vi "GetDisplayProperties.vi"(8 "No Error":errorcluster, 11 "Display ID":T2) -> (0 "Error Out":errorcluster, 3 "PropertiesID":T1)   [LabVIEW 2024, in "SDL3.lvlib" / "Video.lvlib"]
doc: "<B>Summary</B>\nGet the properties associated with a display.\n\n<B>Remarks</B>\nThe following read-only properties are provided by SDL:\n\n- <B>SDL_PROP_DISPLAY_HDR_ENABLED_BOOLEAN</B>: true if the display has HDR headroom above the SDR white point. This is for informational and diagnostic purposes only, as not all platforms provide this information at the display level.\n\nOn KMS/DRM:\n- <B>SDL_PROP_DISPLAY_KMSDRM_PANEL_ORIENTATION_NUMBER</B>: the \"panel orientation\" property for the display in degrees of clockwise rotation. Note that this is provided only as a hint, and the application is responsible for any coordinate transformations needed to conform to the requested display orientation."
uses:
  DisplayID--integer.ctl
  Video.lvlib
  Error/Error.lvlib
  Lib/SDL3-32.dll
  Properties/PropertiesID--integer.ctl
  Properties/Properties.lvlib
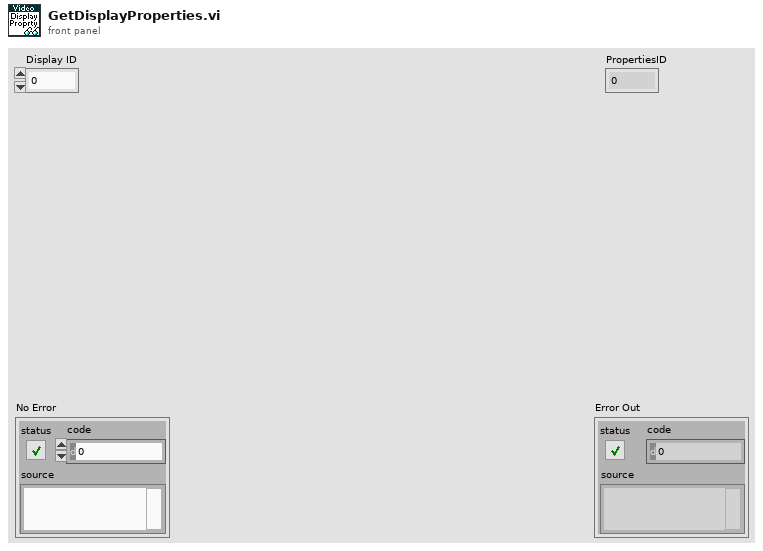
[diagram p1: front panel]
types:
  T1 = typedef "SDL3.lvlib/Properties.lvlib/PropertiesID--integer.ctl" = u32
  T2 = typedef "SDL3.lvlib/Video.lvlib/DisplayID--integer.ctl" = u32
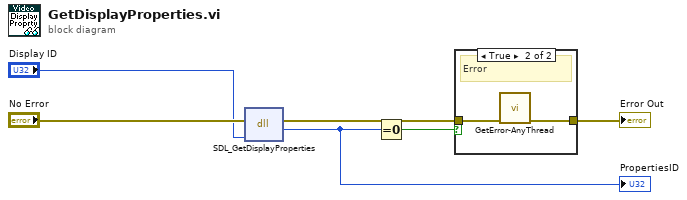
[diagram p0: block diagram]
diagram:
  n1 = dll-call lib="C:/Users/Thomas/Documents/Projects/LV-SDL3/Lib/SDL3-*.*" fn="SDL_GetDisplayProperties"(error in="No Error", "displayID"="Display ID") -> (error out=w3:errorcluster, "return type"=w1:u32)  [unwired: 3 in, 1 out]
  "PropertiesID" <- w1
  n2 = Equal To 0?(x=w1) -> (x = 0?=w2:bool)
  n3 = case shown="True" w2 {
    tunnel: w3 -> [w7 w9]
    tunnel: [w7 w8] -> w5
    frame False {
      # "Ok"
    }
    frame True {
      # "Error"
      n4 = call "GetError-AnyThread.vi"("No Error"=w9) -> ("Error Out"=w8:errorcluster)  [unwired: 10 in]
    }
  }
  "Error Out" <- w5
